vi "Send Is Invalid Waveform Element.vi"(7 "Message Priority (Normal)":T1=enum."Normal", 8 "error in (no error)":errorcluster, 10 "element value (0.0)":dbl format="%.4f", 11 "Message Enqueuer":refnum<class "Message Enqueuer.lvclass">) -> (0 "error out":errorcluster, 3 "Message Enqueuer out":refnum<class "Message Enqueuer.lvclass">)   [LabVIEW 2016, in "CS++Scope.lvlib" / "Is Invalid Waveform Element Msg.lvclass"]
doc: "Sends the <B>CS++Scope.lvlib:Is Invalid Waveform Element Msg.lvclass</B> message.\n\n<B>CS++Scope.lvlib:CS++Scope.lvclass:Is Invalid Waveform Element.vi</B> Description:\n\nAfter the read and fetch waveform VIs execute, each element in the waveform array contains either a voltage or a value indicating that the oscilloscope could not sample a voltage. The driver uses an IEEE defined NaN (Not a Number) value to mark as invalid each element in the waveform array for which the oscilloscope could not sample a voltage. This VI determines whether a value you pass from the waveform array is invalid."
uses:
  Is Invalid Waveform Element Msg.lvclass
  <vilib>/ActorFramework/Message Enqueuer/Message Enqueuer.lvclass
  <vilib>/ActorFramework/Message Enqueuer/Message Priority.ctl
  C:/Program Files (x86)/National Instruments/LabVIEW 2016/vi.lib/ActorFramework/Message/Message.lvclass
  Is Invalid Waveform Element Msg.lvclass/Is Invalid Waveform Element Msg.ctl
  <vilib>/ActorFramework/Message Enqueuer/Message Enqueuer.lvclass/Message Enqueuer.ctl
  <vilib>/ActorFramework/Message Priority Queue/Priority Enqueue.vi
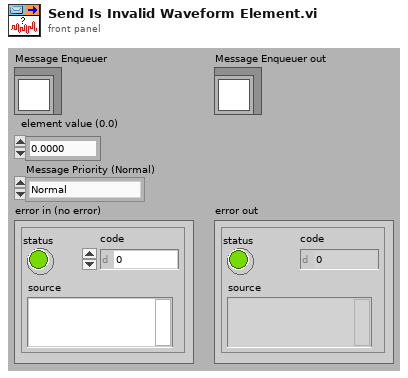
[diagram p1: front panel]
types:
  T1 = typedef "Actor Framework.lvlib/Message Enqueuer.lvclass/Message Priority.ctl" = enum16{"Low", "Normal", "High"}
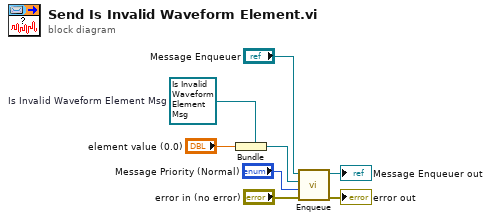
[diagram p0: block diagram]
diagram:
  w2 = refnum<class "Is Invalid Waveform Element Msg.lvclass"> refnum  # Is Invalid Waveform Element Msg
  n1 = Bundle(cluster=w2, "element value (0.0)") -> (w5:refnum<class "Is Invalid Waveform Element Msg.lvclass">)
  n2 = call <vilib>:"Enqueue.vi"("error in (no error)"="error in (no error)", "Message Priority (Normal)"="Message Priority (Normal)", "Message"=w5, "Message Enqueuer in"="Message Enqueuer") -> ("error out"=→"error out":errorcluster, "Message Enqueuer out"=→"Message Enqueuer out":refnum<class "Message Enqueuer.lvclass">)  [unwired: 6 in]
